vi "Sol.vi"(9 "Previous Sol_RaiseDrop":T1, 10 "Joy_L_Buttons":bool[](array[boolean]), 11 "Joy_R_Buttons":bool[](array[boolean])) -> (1 "Sol_RaiseDrop":T1, 3 "Sol_Clamp":T1)   [LabVIEW 2017]
uses:
  <vilib>/Rock Robotics/WPI/Solenoid/WPI_SolenoidValue.ctl
  TypeDefs/joybuttons.ctl
  <vilib>/ptbypt/NI_PtbyPt.lvlib
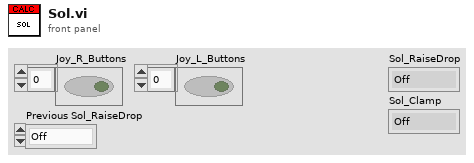
[diagram p1: front panel]
types:
  T1 = typedef "WPI_SolenoidValue.ctl" = enum16{"Off", "On", "Forward", "Reverse"}
  T2 = typedef "joybuttons.ctl" = enum16{"Trigger", "Thumb", "Top3", "Top4", "Top5", "Top6", "Bottom7", "Bottom8", "Bottom9", "Bottom10", "Bottom11", "Bottom12", ""}
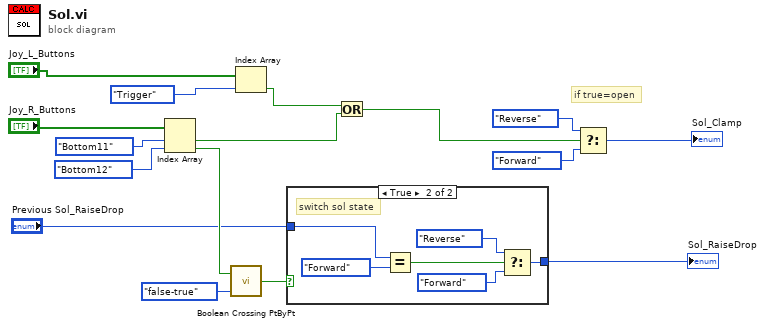
[diagram p0: block diagram]
diagram:
  # "if true=open"
  n1 = Index Array(array="Joy_R_Buttons", index #1=joybuttons."Bottom11" ("Enum"), index #2=joybuttons."Bottom12" ("Enum")) -> (element #1=w2:bool, element #2=w11:bool)
  n2 = call <vilib>:"Boolean Crossing PtByPt.vi"("direction"=enum16{"either", "false-true", "true-false"}."false-true", "input"=w11) -> ("crossing"=w10:bool)  [unwired: 1 in]
  n3 = Index Array(array="Joy_L_Buttons", index=joybuttons."Trigger" ("Enum")) -> (element=w3:bool)
  n4 = case shown="True" w10 {
    tunnel: "Previous Sol_RaiseDrop" -> [w17 w19]
    tunnel: [w17 w18] -> w7
    frame False {
    }
    frame True {
      # "switch sol state"
      n5 = Equal?(x=w19, y=WPI_SolenoidValue."Forward" ("Value")) -> (x = y?=w21:bool)
      n6 = Select(t=WPI_SolenoidValue."Reverse" ("Value"), s=w21, f=WPI_SolenoidValue."Forward" ("Value")) -> (s? t:f=w18:T1)
    }
  }
  "Sol_RaiseDrop" <- w7
  n7 = Or(x=w3, y=w2) -> (x .or. y?=w1:bool)
  n8 = Select(t=WPI_SolenoidValue."Reverse" ("Value"), s=w1, f=WPI_SolenoidValue."Forward" ("Value")) -> (s? t:f=→"Sol_Clamp":T1)
